vi "RSZVB Get Trace Ref Position.vi"(8 "error in (no error)":errorcluster {"code" format="%.0x"}, 9 "Window (Trace) (1)":i32=1, 10 "Window (1)":i32=1, 11 "VISA session":refnum<visa-resource-name>) -> (0 "error out":errorcluster {"code" format="%.0x"}, 2 "Reference Position":dbl format="%^.3e", 3 "dup VISA session":refnum<visa-resource-name>)   [LabVIEW 2011]
doc: "This VI returns the point on the y-axis used as the reference position as a percentage of the length of the y-axis. The reference position is the point on the y-axis which should equal the RLEVel.\n\nNote(s):\n\n(1) Window:\nNumber of an existing diagram area (defined by means of DISPlay:WINDow<Wnd>:STATe ON). \n \n(2) Window (Trace):\nExisting trace number, assigned by means of DISPlay:WINDow<Wnd>:TRACe<WndTr>:FEED.\n\nRemote-control command(s):\nDISPlay:WINDow<Wnd>:TRACe<WndTr>:Y[:SCALe]:RPOSition?"
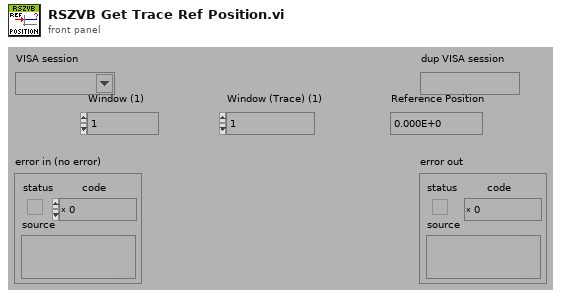
[diagram p1: front panel]
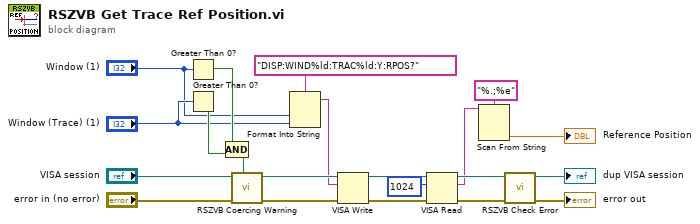
[diagram p0: block diagram]
diagram:
  n1 = Greater Than 0?(x="Window (1)") -> (x > 0?=w15:bool)
  n2 = Greater Than 0?(x="Window (Trace) (1)") -> (x > 0?=w16:bool)
  n3 = Compound Arithmetic op=AND(w15, w16) -> (w18:bool)
  n4 = call "RSZVB Coercing Warning.vi"("In Range?"=w18, "error in (no error)"="error in (no error)", "VISA session"="VISA session") -> ("error out"=w19:errorcluster, "dup VISA session"=w20:refnum<visa-resource-name>)  [unwired: 7 in]
  n5 = Format Into String(format string="DISP:WIND%ld:TRAC%ld:Y:RPOS?", "Window (1)", "Window (Trace) (1)") -> (resulting string=w17:string)  [unwired: 2 in, 1 out]
  n6 = VISA Write(VISA resource name=w20, write buffer=w17, error in (no error)=w19) -> (VISA resource name out=w12:refnum<visa-resource-name>, error out=w14:errorcluster)  [unwired: 1 out]
  n7 = VISA Read(VISA resource name=w12, byte count=u32 1024 ("byte count (0)"), error in (no error)=w14) -> (VISA resource name out=w11:refnum<visa-resource-name>, read buffer=w8:string, error out=w10:errorcluster)  [unwired: 1 out]
  n8 = Scan From String(format string="%.;%e", input string=w8) -> (output 1=→"Reference Position":dbl)  [unwired: 3 in, 3 out]
  n9 = call "RSZVB Check Error.vi"("error in (no error)"=w10, "VISA session"=w11) -> ("error out"=→"error out":errorcluster, "dup VISA session"=→"dup VISA session":refnum<visa-resource-name>)  [unwired: 8 in]
